vi "Get Attributes.vi"(8 "error in (no error)":errorcluster, 11 "ToneCloud in":refnum<class "Tone Cloud.lvclass">) -> (0 "error out":errorcluster, 2 "Attributes":T1, 3 "ToneCloud out":refnum<class "Tone Cloud.lvclass">)   [LabVIEW 2020, in "Tone Cloud.lvclass"]
uses:
  Tone Cloud.lvclass
  Waveform/Attributes.ctl
  Waveform/Waveform.lvclass
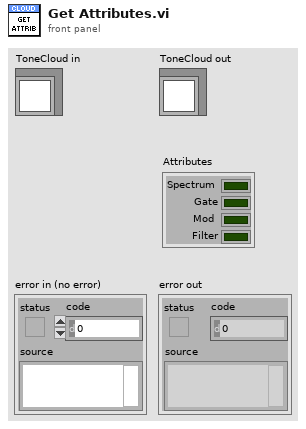
[diagram p1: front panel]
types:
  T1 = typedef "Waveform.lvclass/Attributes.ctl" = cluster{"Spectrum":bool, "Gate":bool, "Mod":bool, "Filter":bool}
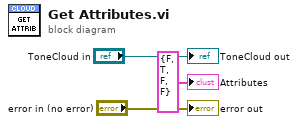
[diagram p0: block diagram]
diagram:
  "error out" <- "error in (no error)"
  "ToneCloud out" <- "ToneCloud in"
  "Attributes" <- T1 {"Spectrum"=FALSE, "Gate"=TRUE, "Mod"=FALSE, "Filter"=FALSE} ("Attributes")
